vi "Autonomous Independent.vi"   [LabVIEW 2013]
doc: "This VI is called when autonomous begins, and will automatically be terminated when autonomous ends. You can carry out timed or sensor driven robot movement independently without needing to return to the caller."
uses:
  <vilib>/Rock Robotics/WPI/Solenoid/WPI_SolenoidValue.ctl
  <vilib>/Rock Robotics/WPI/RobotDrive/WPI_RobotDriveGetSetRefNum.vi
  <vilib>/Rock Robotics/WPI/Solenoid/Deprecated/WPI_SolenoidGetBool.vi
  <vilib>/Rock Robotics/WPI/Solenoid/WPI_SolenoidSetEnum.vi
panel:
  # "Be sure to right-click and choose Data Operations>>Make Current Value default if you want to save the array values with the VI"
types:
  T1 = typedef "WPI_RobotDriveDevRef.ctl" = cluster{"DevStatus":errorcluster, "Motors[]":T2[], "Square Inputs":bool, "Max Output":dbl, "Isochronous":bool}
  T2 = typedef "WPI_MotorControlDeviceRef.ctl" = cluster{"DeviceStatus":errorcluster, "Type":enum16{"PWM", "CAN"}, "PWM":cluster{"Digital Module":T3, "PWM Channel":T4, "DeadBand":T5}, "CAN":cluster{"Device Number":u8, "Control Mode":T6, "Semaphore":T7, "Max Vout":dbl}, "Invert":bool, "TransformRef":T8, "InvTransformRef":T8}
  T3 = typedef "FPGA_TypedefDigitalModule.ctl" = enum16{"Digital Module 1", "Digital Module 2"}
  T4 = typedef "FPGA_DIOPWMChannel.ctl" = enum8{"PWM 1", "PWM 2", "PWM 3", "PWM 4", "PWM 5", "PWM 6", "PWM 7", "PWM 8", "PWM 9", "PWM 10", "Invalid"}
  T5 = typedef "WPI_PWMDeadband.ctl" = cluster{"Name":string, "maxPositivePwm":i32, "minPositivePwm":i32, "centerPwm":i32, "maxNegativePwm":i32, "minNegativePwm":i32, "angularRange":u16}
  T6 = typedef "WPI_CANJaguar_ControlMode.ctl" = enum8{"Percent VBus", "Current", "Speed", "Position", "Voltage"}
  T7 = typedef "Semaphore RefNum" = refnum<k1>
  T8 = typedef "WPI_PWMTransform_ConPane.ctl" = refnum<vi>
  T9 = typedef "WPI_SolenoidDevRef.ctl" = cluster{"DevStatus":errorcluster, "Solenoid Module":T10, "Forward Solenoid Channel":T11, "Reverse Solenoid Channel":T11}
  T10 = typedef "FPGA_TypedefSolenoidModule.ctl" = enum16{"Solenoid Module 1", "Solenoid Module 2"}
  T11 = typedef "WPI_SolenoidChannel.ctl" = enum8{"Solenoid 1", "Solenoid 2", "Solenoid 3", "Solenoid 4", "Solenoid 5", "Solenoid 6", "Solenoid 7", "Solenoid 8", "Invalid"}
  T12 = typedef "WPI_SolenoidValue.ctl" = enum16{"Off", "On", "Forward", "Reverse"}
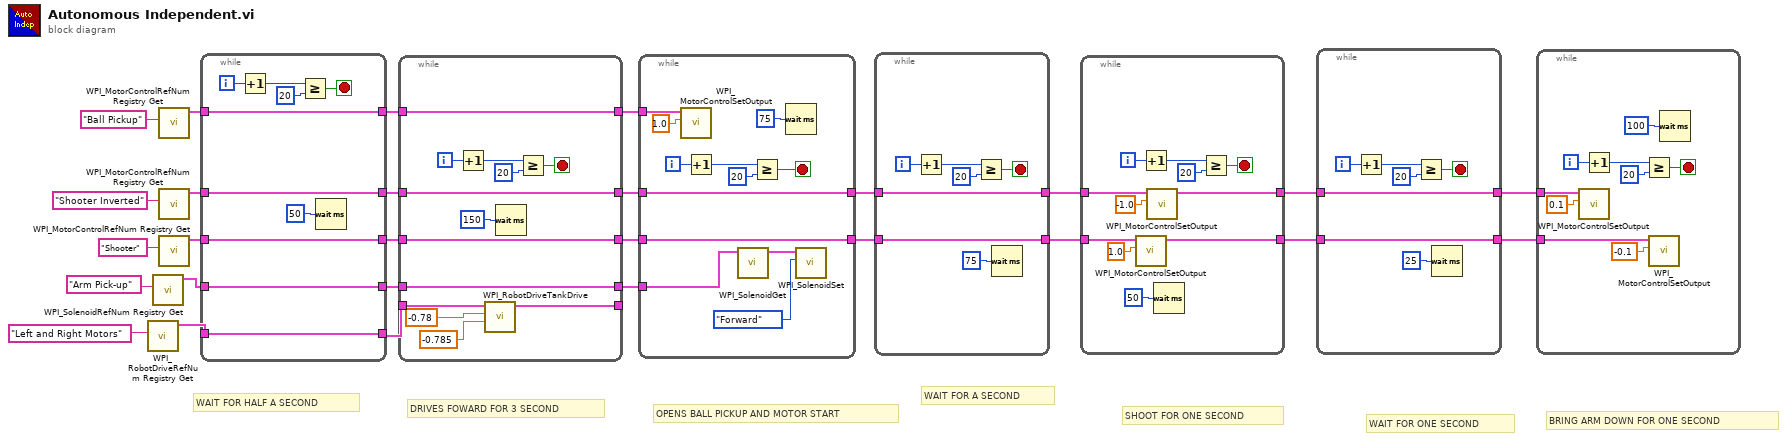
[diagram p0: block diagram]
diagram:
  # "WAIT FOR A SECOND"
  # "WAIT FOR ONE SECOND"
  # "BRING ARM DOWN FOR ONE SECOND"
  # "WAIT FOR HALF A SECOND"
  # "SHOOT FOR ONE SECOND"
  # "OPENS BALL PICKUP AND MOTOR START"
  # "DRIVES FOWARD FOR 3 SECOND"
  n1 = call <vilib>:"WPI_RobotDriveRefNum Registry Get.vi"("refnum name"="Left and Right Motors") -> ("RobotDriveDevRef"=w24:T1)  [unwired: 9 in, 1 out]
  n2 = call <vilib>:"WPI_SolenoidRefNum Registry Get.vi"("refnum name"="Arm Pick-up") -> ("SolenoidDevRef"=w25:T9)  [unwired: 9 in, 1 out]
  n3 = call <vilib>:"WPI_MotorControlRefNum Registry Get.vi"("refnum name"="Ball Pickup") -> ("MotorControlDevRef"=w18:T2)  [unwired: 9 in, 1 out]
  n4 = call <vilib>:"WPI_MotorControlRefNum Registry Get.vi"("refnum name"="Shooter Inverted") -> ("MotorControlDevRef"=w21:T2)  [unwired: 9 in, 1 out]
  n5 = call <vilib>:"WPI_MotorControlRefNum Registry Get.vi"("refnum name"="Shooter") -> ("MotorControlDevRef"=w20:T2)  [unwired: 9 in, 1 out]
  n6 = while {
    tunnel: w25 -> [w29]
    tunnel: [w37] -> w1
    tunnel: w24 -> [w37]
    tunnel: w21 -> [w31]
    tunnel: [w31] -> w16
    tunnel: w20 -> [w30]
    tunnel: [w30] -> w17
    tunnel: w18 -> [w28]
    tunnel: [w29] -> w13
    tunnel: [w28] -> w11
    i -> [w34]
    stop <- w33 stop-if-true
    n7 = Increment(x=w34) -> (x+1=w35:i32)
    n8 = Greater Or Equal?(x=w35, y=20) -> (x >= y?=w33:bool)
    n9 = Wait (ms)(milliseconds to wait=u32 50) -> ()  [unwired: 1 out]
  }
  n10 = while {
    tunnel: w1 -> [w50]
    tunnel: [w43] -> _
    tunnel: w16 -> [w41]
    tunnel: [w41] -> w15
    tunnel: w17 -> [w40]
    tunnel: [w40] -> w14
    tunnel: w13 -> [w39]
    tunnel: [w39] -> w12
    tunnel: [w38] -> w10
    tunnel: w11 -> [w38]
    i -> [w48]
    stop <- w45 stop-if-true
    n11 = Increment(x=w48) -> (x+1=w47:i32)
    n12 = call <vilib>:"WPI_RobotDriveTankDrive.vi"("Right axis value"=-0.785 ("Y axis value"), "Left axis value"=-0.78 ("X axis value"), "RobotDriveDevRef"=w50) -> ("RobotDriveDevRef"=w43:T1)  [unwired: 6 in, 2 out]
    n13 = Wait (ms)(milliseconds to wait=u32 150) -> ()  [unwired: 1 out]
    n14 = Greater Or Equal?(x=w47, y=20) -> (x >= y?=w45:bool)
  }
  n15 = while {
    tunnel: [w62] -> w3
    tunnel: w15 -> [w62]
    tunnel: [w61] -> w4
    tunnel: w14 -> [w61]
    tunnel: w12 -> [w53]
    tunnel: w10 -> [w51]
    i -> [w59]
    stop <- w57 stop-if-true
    n16 = call <vilib>:"WPI_MotorControlSetOutput.vi"("Output"=1.0, "MotorControlDevRef"=w51) -> ()  [unwired: 7 in, 3 out]
    n17 = Increment(x=w59) -> (x+1=w60:i32)
    n18 = call-poly <vilib>:"WPI_SolenoidGet.vi"("SolenoidDevRef"=w53) -> ("SolenoidDevRef"=w54:T9)  [unwired: 8 in, 2 out]
    n19 = Greater Or Equal?(x=w60, y=20) -> (x >= y?=w57:bool)
    n20 = Wait (ms)(milliseconds to wait=u32 75) -> ()  [unwired: 1 out]
    n21 = call-poly <vilib>:"WPI_SolenoidSet.vi"("Value"=WPI_SolenoidValue."Forward", "SolenoidDevRef"=w54) -> ()  [unwired: 8 in, 2 out]
  }
  n22 = while {
    tunnel: [w64] -> w5
    tunnel: w4 -> [w64]
    tunnel: w3 -> [w63]
    tunnel: [w63] -> w2
    i -> [w69]
    stop <- w66 stop-if-true
    n23 = Increment(x=w69) -> (x+1=w68:i32)
    n24 = Greater Or Equal?(x=w68, y=20) -> (x >= y?=w66:bool)
    n25 = Wait (ms)(milliseconds to wait=u32 75) -> ()  [unwired: 1 out]
  }
  n26 = while {
    tunnel: [w73] -> w9
    tunnel: [w72] -> w8
    tunnel: w5 -> [w71]
    tunnel: w2 -> [w70]
    i -> [w78]
    stop <- w77 stop-if-true
    n27 = call <vilib>:"WPI_MotorControlSetOutput.vi"("Output"=1.0, "MotorControlDevRef"=w71) -> ("MotorControlDevRef"=w72:T2)  [unwired: 7 in, 2 out]
    n28 = Increment(x=w78) -> (x+1=w80:i32)
    n29 = call <vilib>:"WPI_MotorControlSetOutput.vi"("Output"=-1.0, "MotorControlDevRef"=w70) -> ("MotorControlDevRef"=w73:T2)  [unwired: 7 in, 2 out]
    n30 = Wait (ms)(milliseconds to wait=u32 50) -> ()  [unwired: 1 out]
    n31 = Greater Or Equal?(x=w80, y=20) -> (x >= y?=w77:bool)
  }
  n32 = while {
    tunnel: [w82] -> w6
    tunnel: w9 -> [w82]
    tunnel: [w81] -> w7
    tunnel: w8 -> [w81]
    i -> [w85]
    stop <- w84 stop-if-true
    n33 = Increment(x=w85) -> (x+1=w87:i32)
    n34 = Greater Or Equal?(x=w87, y=20) -> (x >= y?=w84:bool)
    n35 = Wait (ms)(milliseconds to wait=u32 25) -> ()  [unwired: 1 out]
  }
  n36 = while {
    tunnel: w7 -> [w89]
    tunnel: w6 -> [w88]
    i -> [w94]
    stop <- w93 stop-if-true
    n37 = call <vilib>:"WPI_MotorControlSetOutput.vi"("Output"=0.1, "MotorControlDevRef"=w88) -> ()  [unwired: 7 in, 3 out]
    n38 = Increment(x=w94) -> (x+1=w95:i32)
    n39 = Greater Or Equal?(x=w95, y=20) -> (x >= y?=w93:bool)
    n40 = call <vilib>:"WPI_MotorControlSetOutput.vi"("Output"=-0.1, "MotorControlDevRef"=w89) -> ()  [unwired: 7 in, 3 out]
    n41 = Wait (ms)(milliseconds to wait=u32 100) -> ()  [unwired: 1 out]
  }
